vi "DSF.Engine.Interface.RT FIFO.Write.vi"   [LabVIEW 2017, in "Data Sharing Framework Engine.lvlib" / "DSF.Engine.Interface.lvclass"]
uses:
  DSF.Engine.Interface.lvclass
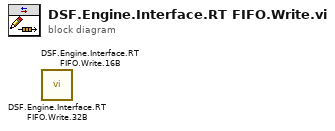
[diagram p0: block diagram]
diagram:
  n1 = call "DSF.Engine.Interface.RT FIFO.Write.32B.vi"() -> ()  [unwired: 9 in, 3 out]
  n2 = call "DSF.Engine.Interface.RT FIFO.Write.16B.vi"() -> ()  [unwired: 9 in, 3 out]
